vi "TDC_修正后数据计算.vi"(1 "细计数输入2":dbl[](array[numeric]), 2 "细计数输入1":dbl[](array[numeric]), 3 "粗计数":dbl[](array[numeric])) -> (0 "分布谱":dbl[](graph))   [LabVIEW 2014]
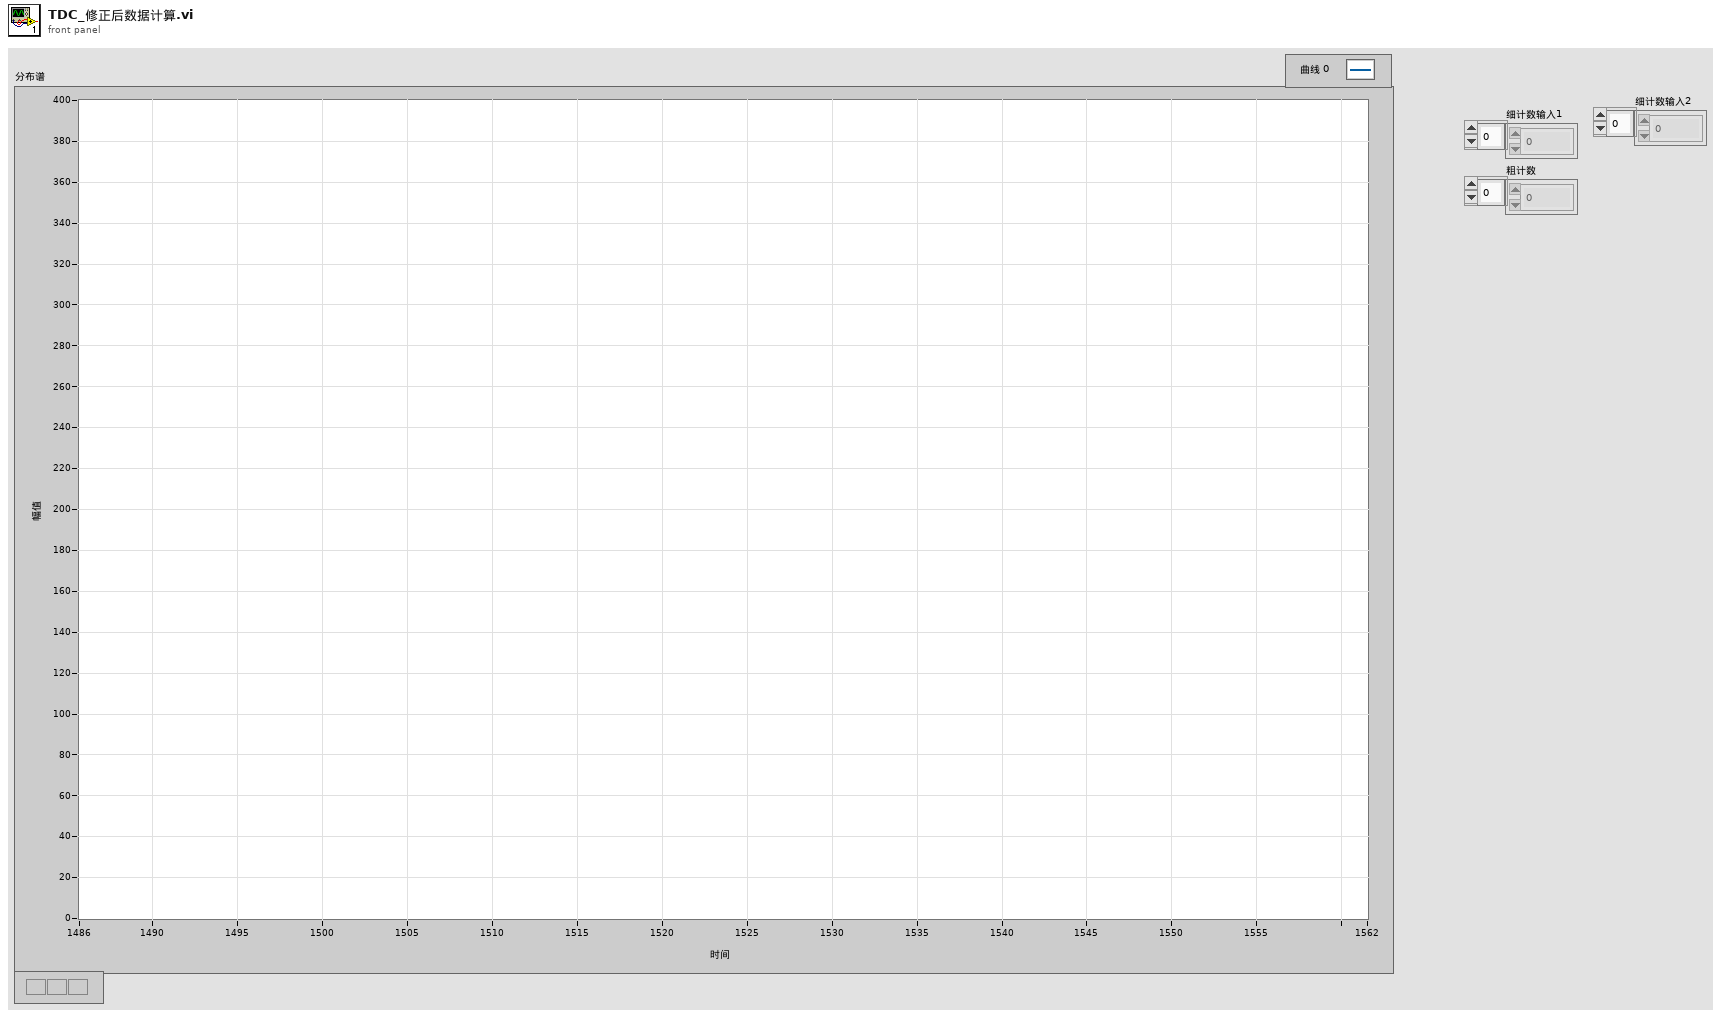
[diagram p1: front panel]
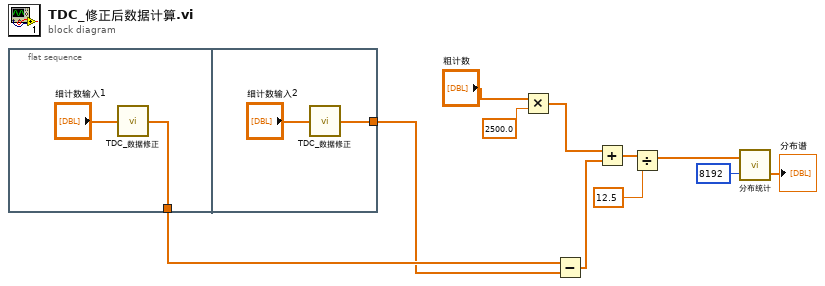
[diagram p0: block diagram]
diagram:
  n1 = flat-sequence {
    tunnel: [w12] -> w4
    tunnel: [w14] -> w3
    frame #0 {
      n2 = call "TDC_数据修正.vi"("细计数输入"="细计数输入1") -> ("修正后的细计数"=w12:dbl[])
    }
    frame #1 {
      n3 = call "TDC_数据修正.vi"("细计数输入"="细计数输入2") -> ("修正后的细计数"=w14:dbl[])
    }
  }
  n4 = Multiply(x="粗计数", y=2500.0) -> (x*y=w2:dbl[])
  n5 = Subtract(x=w4, y=w3) -> (x-y=w11:dbl[])
  n6 = Add(x=w2, y=w11) -> (x+y=w7:dbl[])
  n7 = Divide(x=w7, y=12.5) -> (x/y=w6:dbl[])
  n8 = call "分布统计.vi"("道数"=8192, "数组"=w6) -> ("分布谱"=→"分布谱":dbl[])  [unwired: 1 out]
